vi "text to number.vi"(1 "text":string) -> (0 "number":dbl format="%#_10g")   [LabVIEW 2017]
doc: "This vi identifies variables appear in durations, and convert the string format durations to real number durations"
uses:
  globals/Global variables.vi
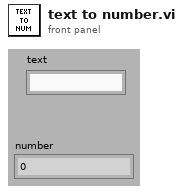
[diagram p1: front panel]
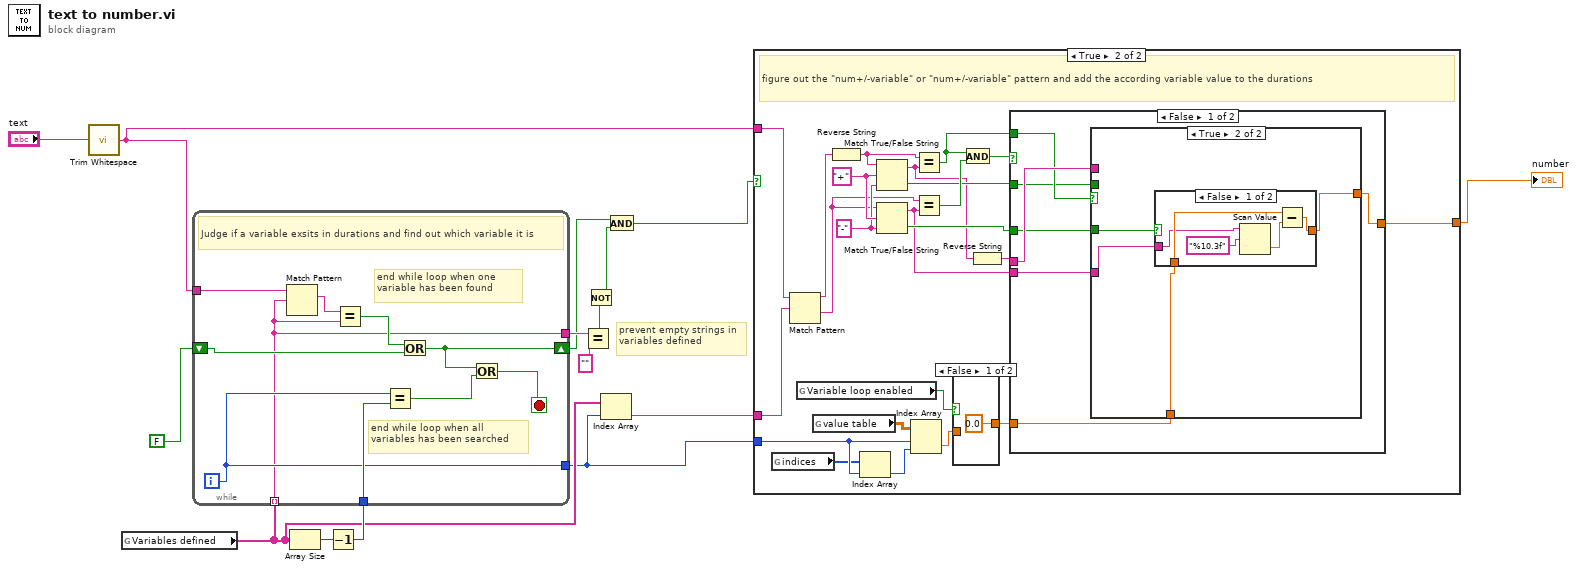
[diagram p0: block diagram]
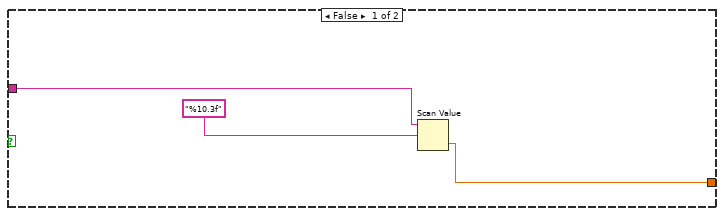
[diagram p2: hidden frame]
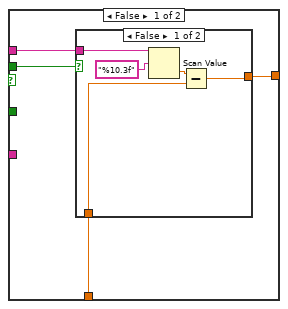
[diagram p4: hidden frame]
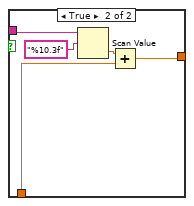
[diagram p5: hidden frame]
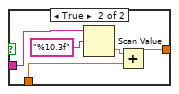
[diagram p6: hidden frame]
diagram:
  # "prevent empty strings in variables defined"
  n1 = call <vilib>:"Trim Whitespace.vi"("string"="text") -> ("trimmed string"=w15:string)  [unwired: 1 in]
  n2 = global read "Global variables.vi" "Variables defined"() -> (w11:string[])
  n3 = Array Size(array=w11) -> (size(s)=w13:i32)
  n4 = Decrement(x=w13) -> (x-1=w12:i32)
  n5 = while {
    tunnel: w11 -> [w16] mode=indexing
    tunnel: w15 -> [w25]
    shift-right: [w21] -> w4
    shift-left: FALSE -> [w23]
    tunnel: w12 -> [w22]
    tunnel: [w18] -> w9
    tunnel: [w16] -> w8
    i -> [w18]
    stop <- w19 stop-if-true
    # "end while loop when one variable has been found"
    # "end while loop when all variables has been searched"
    # "Judge if a variable exsits in durations and find out which variable it is"
    n6 = Match Pattern(string=w25, regular expression=w16) -> (match substring=w17:string)  [unwired: 1 in, 3 out]
    n7 = Equal?(x=w17, y=w16) -> (x = y?=w24:bool)
    n8 = Equal?(x=w18, y=w22) -> (x = y?=w20:bool)
    n9 = Or(x=w24, y=w23) -> (x .or. y?=w21:bool)
    n10 = Or(x=w21, y=w20) -> (x .or. y?=w19:bool)
  }
  n11 = Equal?(x=w8, y="") -> (x = y?=w6:bool)
  n12 = Not(x=w6) -> (.not. x?=w5:bool)
  n13 = Index Array(array=w11, index=w9) -> (element=w10:string)
  n14 = And(x=w4, y=w5) -> (x .and. y?=w3:bool)
  n15 = case shown="True" w3 {
    tunnel: [w28 w40] -> w1
    tunnel: w15 -> [w26 w38]
    tunnel: w10 -> [_ w39]
    tunnel: w9 -> [_ w34]
    frame False {
      n16 = Scan Value(string=w26, format string="%10.3f") -> (value=w28:dbl)  [unwired: 1 in, 1 out]
    }
    frame True {
      w50 = "-" ("regular expression")
      w51 = "+" ("regular expression")
      # "figure out the \"num+/-variable\" or \"num+/-variable\" pattern and add the according variable value to the durations"
      n17 = global read "Global variables.vi" "indices"() -> (w33:i32[])
      n18 = Match Pattern(string=w38, regular expression=w39) -> (before substring=w37:string, after substring=w36:string)  [unwired: 1 in, 2 out]
      n19 = global read "Global variables.vi" "Variable loop enabled"() -> (w31:bool)
      n20 = global read "Global variables.vi" "value table"() -> (w35:dbl[][])
      n21 = Reverse String(1:w37) -> (0:w48:string)
      n22 = Index Array(array=w33, index=w34) -> (element=w32:i32)
      n23 = Match True/False String(2:w50, 3:w51, 4:w48) -> (0:w46:bool, 1:w41:string)
      n24 = Match True/False String(2:w50, 3:w51, 4:w36) -> (0:w44:bool, 1:w43:string)
      n25 = Index Array(array=w35, index (row)=w34, index (col)=w32) -> (element=w30:dbl)
      n26 = Equal?(x=w48, y=w41) -> (x = y?=w45:bool)
      n27 = Equal?(x=w36, y=w43) -> (x = y?=w49:bool)
      n28 = case shown="False" w31 {
        tunnel: w30 -> [_ w53]
        tunnel: [0.0 ("Numeric") w53] -> w29
        frame False {
        }
        frame True {
        }
      }
      n29 = And(x=w45, y=w49) -> (x .and. y?=w47:bool)
      n30 = Reverse String(1:w41) -> (0:w42:string)
      n31 = case shown="False" w47 {
        tunnel: [w58 w89] -> w40
        tunnel: w46 -> [w56 _]
        tunnel: w42 -> [w60 _]
        tunnel: w29 -> [w59 w89]
        tunnel: w45 -> [w57 _]
        tunnel: w44 -> [w55 _]
        tunnel: w43 -> [w54 _]
        frame False {
          n32 = case shown="True" w57 {
            tunnel: w60 -> [w64 _]
            tunnel: w59 -> [w63 w78]
            tunnel: [w62 w77] -> w58
            tunnel: w56 -> [w61 _]
            tunnel: w55 -> [_ w76]
            tunnel: w54 -> [_ w75]
            frame False {
              n33 = case shown="False" w61 {
                tunnel: w64 -> [w66 w72]
                tunnel: w63 -> [w67 w71]
                tunnel: [w65 w70] -> w62
                frame False {
                  n34 = Scan Value(string=w66, format string="%10.3f") -> (value=w69:dbl)  [unwired: 1 in, 1 out]
                  n35 = Subtract(x=w69, y=w67) -> (x-y=w65:dbl)
                }
                frame True {
                  n36 = Scan Value(string=w72, format string="%10.3f") -> (value=w73:dbl)  [unwired: 1 in, 1 out]
                  n37 = Add(x=w73, y=w71) -> (x+y=w70:dbl)
                }
              }
            }
            frame True {
              n38 = case shown="False" w76 {
                tunnel: w78 -> [w82 w87]
                tunnel: [w80 w85] -> w77
                tunnel: w75 -> [w79 w84]
                frame False {
                  n39 = Scan Value(string=w79, format string="%10.3f") -> (value=w81:dbl)  [unwired: 1 in, 1 out]
                  n40 = Subtract(x=w82, y=w81) -> (x-y=w80:dbl)
                }
                frame True {
                  n41 = Scan Value(string=w84, format string="%10.3f") -> (value=w86:dbl)  [unwired: 1 in, 1 out]
                  n42 = Add(x=w86, y=w87) -> (x+y=w85:dbl)
                }
              }
            }
          }
        }
        frame True {
        }
      }
    }
  }
  "number" <- w1
